vi "DQMH Get Module Type.vi"(8 "error in":errorcluster, 11 "Module Path":path) -> (0 "error out":errorcluster, 3 "Module Types":T1)   [LabVIEW 2020, in "hse-dqmh.lvlib"]
doc: "Returns the type (singleton or cloneable) of the module in <b>Module Path</b>\n\n____\nHAMPEL SOFTWARE ENGINEERING v3.8.0 (2023-12-18 14:41)"
uses:
  hse-dqmh.lvlib
  Controls/Module Types.ctl
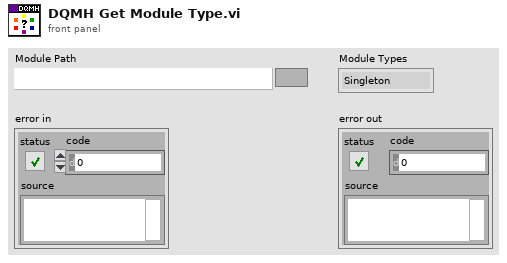
[diagram p1: front panel]
types:
  T1 = typedef "hse-dqmh.lvlib/Module Types.ctl" = enum16{"Singleton", "Cloneable"}
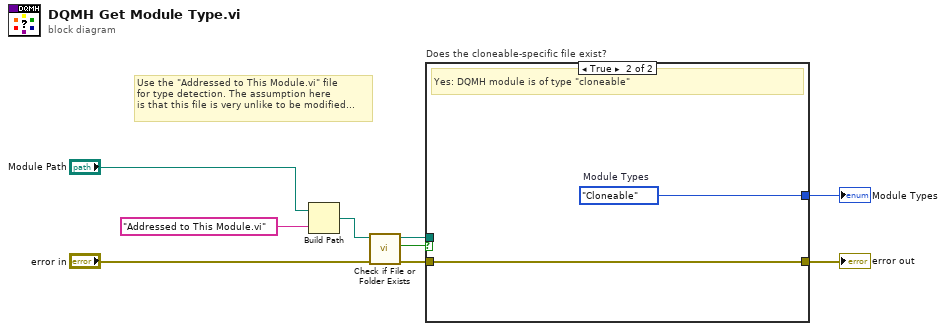
[diagram p0: block diagram]
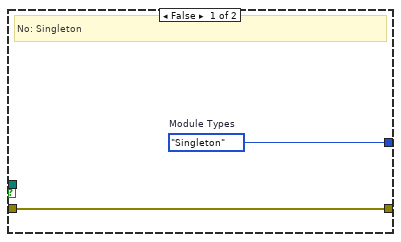
[diagram p2: hidden frame]
diagram:
  # "Use the \"Addressed to This Module.vi\" file\nfor type detection. The assumption here\nis that this file is very unlike to be modified..."
  n1 = Build Path(base path="Module Path", name or relative path="Addressed to This Module.vi") -> (appended path=w2:path)
  n2 = call <vilib>:"Check if File or Folder Exists.vi"("error in (no error)"="error in", "path"=w2) -> ("error out"=w6:errorcluster, "file or folder exists?"=w1:bool, "dup path"=w4:path)  [unwired: 7 in]
  n3 = case "Does the cloneable-specific file exist?" shown="True" w1 {
    tunnel: [w11 w13] -> w5
    tunnel: w4 -> [_ _]
    tunnel: [w10 w12] -> w3
    tunnel: w6 -> [w11 w13]
    frame False {
      w10 = Module_Types."Singleton"  # Module Types
      # "No: Singleton"
    }
    frame True {
      w12 = Module_Types."Cloneable"  # Module Types
      # "Yes: DQMH module is of type \"cloneable\""
    }
  }
  "error out" <- w5
  "Module Types" <- w3
